vi "Band Phase (CPM).vi"(0 "Cross phase [degrees]":cluster{"f0":dbl, "df":dbl, "phase":sgl[]}, 5 "Start":dbl, 7 "Stop":dbl, 11 "error in (no error)":errorcluster) -> (6 "Phase (deg)":sgl, 15 "error out":errorcluster)   [LabVIEW 2017, in "VibrationAnalysisFunctions.lvlib"]
uses:
  <vilib>/addons/InsightCM/Utilities/Analysis/Vibration/VibrationAnalysisFunctions.lvlib
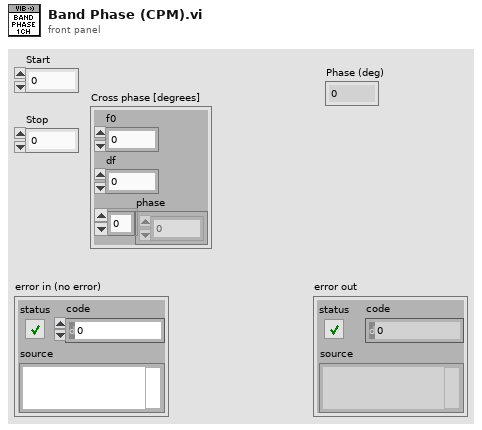
[diagram p1: front panel]
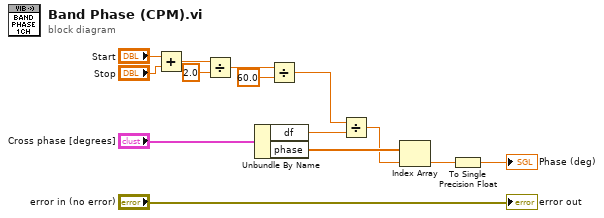
[diagram p0: block diagram]
diagram:
  n1 = Add(x="Start", y="Stop") -> (x+y=w5:dbl)
  n2 = Divide(x=w5, y=2.0) -> (x/y=w3:dbl)
  n3 = Unbundle By Name("Cross phase [degrees]") -> ("df"=w2:dbl, "phase"=w10:sgl[])
  n4 = Divide(x=w3, y=60.0) -> (x/y=w1:dbl)
  n5 = Divide(x=w1, y=w2) -> (x/y=w8:dbl)
  n6 = Index Array(array=w10, index=w8) -> (element=w9:sgl)
  n7 = To Single Precision Float(number=w9) -> (single precision float=→"Phase (deg)":sgl)
  "error out" <- "error in (no error)"
